vi "Set ID.vi"(10 "ID":i32, 11 "Interface in":refnum<class "Interface.lvclass">) -> (3 "Interface out":refnum<class "Interface.lvclass">)   [LabVIEW 2019, in "DSF Core.lvlib" / "Interface.lvclass"]
uses:
  Interface.lvclass
  Interface.lvclass/Interface.ctl
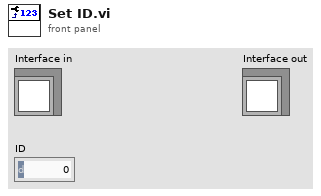
[diagram p1: front panel]
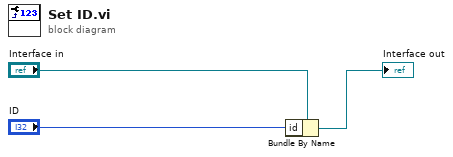
[diagram p0: block diagram]
diagram:
  n1 = Bundle By Name(cluster="Interface in", "id"="ID") -> (→"Interface out":refnum<class "Interface.lvclass">)
